vi "SelectMenu3.vi"(6 "Click Type":T1, 7 "Id":string, 8 "Point":T3, 9 "Item Index":u32, 10 "XRef":refnum<vi>, 11 "State In":T2={"Input Type"=variant(dbl 0.0), "Selection"=0, "Element Names"=[], "Type Strings"=[], "Element Types"=[]}) -> (0 "Reply":string[](array[string]), 3 "State Out":T2={"Input Type"=variant(dbl 0.0), "Selection"=0, "Element Names"=[], "Type Strings"=[], "Element Types"=[]})   [LabVIEW 2015, in "Construct-Tagged-Union.xnode"]
doc: "This ability VI is called after the user selects an item from a portion of the menu defined during BuildMenu. Click Type is the type of click that led to the building of the menu whose selection is being handled by this VI. ItemIndex is the index of the element in the array used when you specified the popup menu. Id is the id you associated with the item in BuildMenu3. Point is the location where the user clicked to build the menu relative to the top-left corner of the XNode. You can display a dialog in response to a user selection if you wish. Use Reply to inform LabVIEW of any actions it needs to take.\n\nDefault behavior: None.\n\nThis ability provides UI and OS messages are handled.\n\nSee also: BuildMenu3"
uses:
  Construct-Tagged-Union.xnode
  State.ctl
  <vilib>/XNodeSupport/XNodePoint.ctl
  <vilib>/XNodeSupport/XNodeInt.ctl
  <vilib>/XNodeSupport/XNodeClickTypes.ctl
  <vilib>/XNodeSupport/NI_XNodeSupport.lvlib
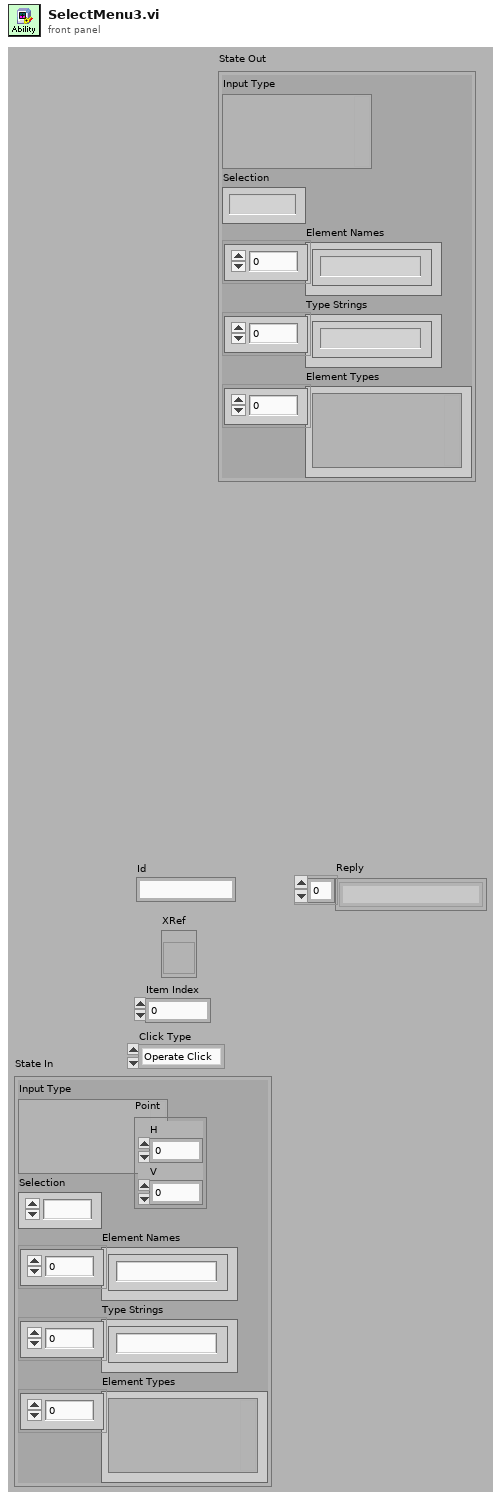
[diagram p1: front panel]
types:
  T1 = typedef "NI_XNodeSupport.lvlib/XNodeClickTypes.ctl" = enum32{"Operate Click", "Popup Click"}
  T2 = typedef "Construct-Tagged-Union.xnode/State.ctl" = cluster{"Input Type":variant, "Selection":i32, "Element Names":string[], "Type Strings":string[], "Element Types":variant[]}
  T3 = typedef "NI_XNodeSupport.lvlib/XNodePoint.ctl" = cluster{"H":T4, "V":T4}
  T4 = typedef "NI_XNodeSupport.lvlib/XNodeInt.ctl" = i32
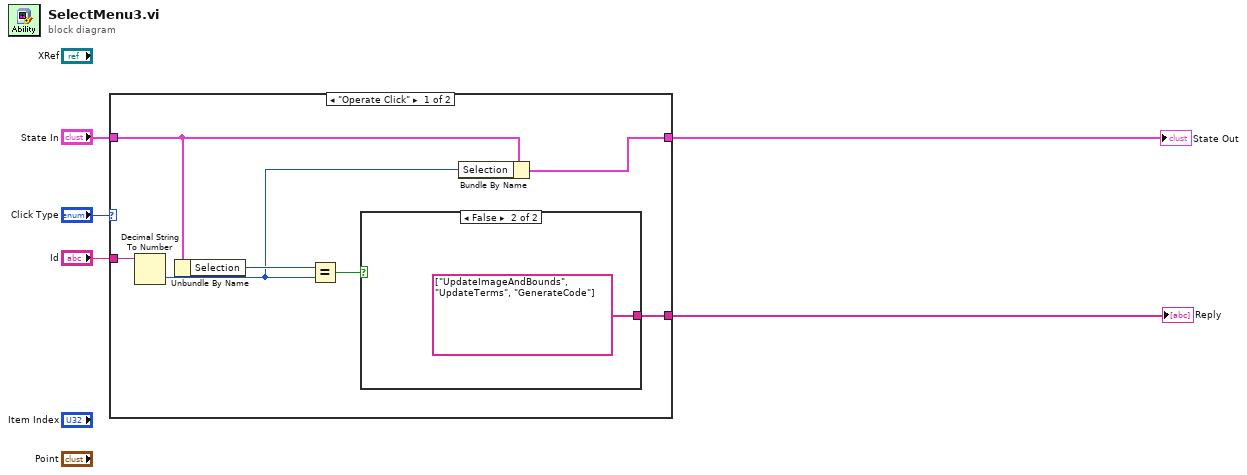
[diagram p0: block diagram]
diagram:
  n1 = case shown="\"Operate Click\"" "Click Type" {
    tunnel: [w12 w14] -> w1
    tunnel: "State In" -> [w10 w14]
    tunnel: "Id" -> [w11 _]
    tunnel: [w6 _] -> w2
    frame "Operate Click" {
      n2 = Decimal String To Number(string=w11) -> (number=w8:i32)  [unwired: 2 in, 1 out]
      n3 = Unbundle By Name(w10) -> ("Selection"=w9:i32)
      n4 = Equal?(x=w9, y=w8) -> (x = y?=w7:bool)
      n5 = case shown="False" w7 {
        tunnel: [_ string[] ["UpdateImageAndBounds", "UpdateTerms", "GenerateCode"] ("Reply")] -> w6
        frame True {
        }
        frame False {
        }
      }
      n6 = Bundle By Name(cluster=w10, "Selection"=w8) -> (w12:T2)
    }
    frame "Popup Click" {
    }
  }
  "State Out" <- w1
  "Reply" <- w2
